vi "Create Debug Text File.vi"(8 "error in (no error)":errorcluster, 10 "text":string, 11 "filename":path) -> (0 "error out":errorcluster, 3 "file path out":path)   [LabVIEW 2020, in "RxnRover.lvlib" / "File IO.lvlib"]
doc: "VI Meant to help the debugging process, allows you to create a .txt file with a given name and given text data at %USER%\\AppData\\Local\\RxnRover\\Debug\\filename.txt"
uses:
  File IO.lvlib
  AppData Utilities/LocalAppData Utilities.lvlib
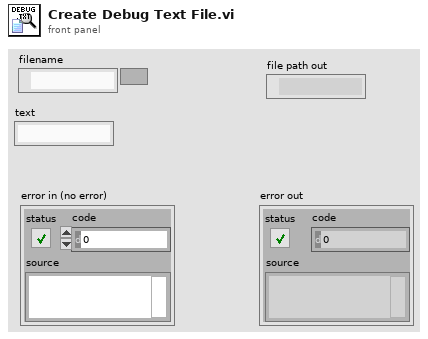
[diagram p1: front panel]
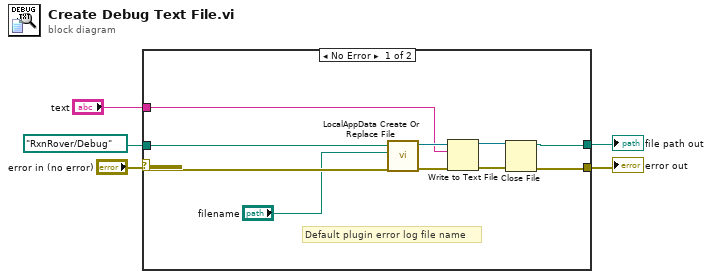
[diagram p0: block diagram]
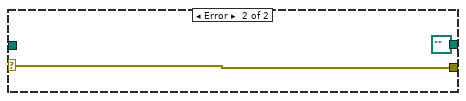
[diagram p2: hidden frame]
diagram:
  n1 = case shown="No Error" "error in (no error)" {
    selector: "error in (no error)" -> [w14 w17]
    tunnel: path "RxnRover/Debug" ("relative file path") -> [w15 _]
    tunnel: [w13 w17] -> w5
    tunnel: [w12 path "" ("path")] -> w3
    tunnel: "text" -> [w6 _]
    frame No Error {
      # "Default plugin error log file name"
      n2 = call "LocalAppData Create Or Replace File.vi"("error in (no error)"=w14, "filename"="filename", "relative file path"=w15) -> ("error out"=w8:errorcluster, "Byte Stream File out"=w7:refnum<file>)  [unwired: 7 in]
      n3 = Write to Text File(file (use dialog)=w7, text=w6, error in=w8) -> (refnum out=w9:refnum<file>, error out=w10:errorcluster)  [unwired: 1 in, 1 out]
      n4 = Close File(refnum=w9, error in=w10) -> (path=w12:path, error out=w13:errorcluster)
    }
    frame Error {
    }
  }
  "error out" <- w5
  "file path out" <- w3
